vi "Copy PPLs to Includes.vi"(5 "Files Generated by Build":path[](array[path]), 6 "Top Level/Always Included VIs":path[](array[path]), 7 "Destination Path":path, 8 "error in (no error)":errorcluster, 9 "Target Name":string, 10 "Build Specification Name":string, 11 "Project Path":path) -> (0 "error out":errorcluster)   [LabVIEW 2020]
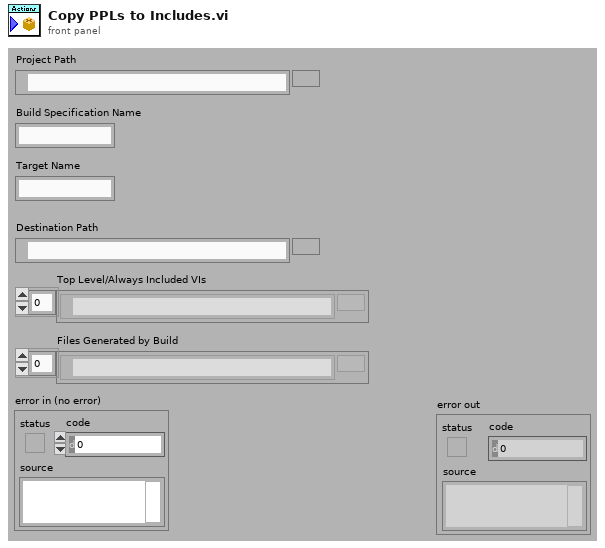
[diagram p1: front panel]
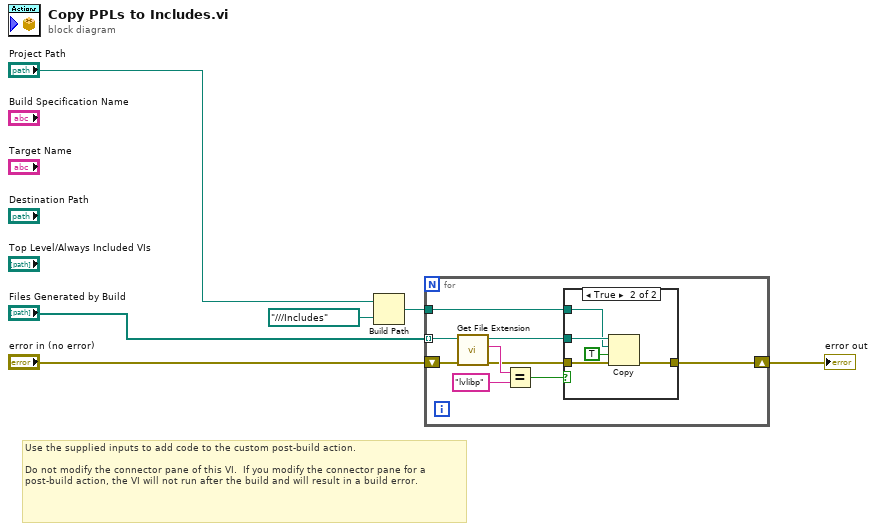
[diagram p0: block diagram]
diagram:
  # "Use the supplied inputs to add code to the custom post-build action.\n\nDo not modify the connector pane of this VI.  If you modify the connector pane for a post-build action, the VI will not run after the build and will result in a build error."
  n1 = Build Path(base path="Project Path", name or relative path=path "../../../Includes") -> (appended path=w1:path)
  n2 = for {
    shift-right: [w10] -> w5
    shift-left: "error in (no error)" -> [w15]
    tunnel: "Files Generated by Build" -> [w14] mode=indexing
    tunnel: w1 -> [w7]
    n3 = call <vilib>:"Get File Extension.vi"("error in (no error)"=w15, "file"=w14) -> ("error out"=w11:errorcluster, "lowercase file extension"=w13:string, "dup file"=w9:path)  [unwired: 5 in, 2 out]
    n4 = Equal?(x=w13, y="lvlibp") -> (x = y?=w8:bool)
    n5 = case shown="True" w8 {
      tunnel: w11 -> [w16 w21]
      tunnel: [w16 w20] -> w10
      tunnel: w9 -> [_ w18]
      tunnel: w7 -> [_ w17]
      frame False {
      }
      frame True {
        n6 = Copy(8:w21, 9:TRUE ("overwrite (F)"), 10:w17, 11:w18) -> (0:w20:errorcluster)  [unwired: 1 in, 2 out]
      }
    }
  }
  "error out" <- w5
